vi "Decode FST200 Direction Response.vi"(10 "Direction Modbus Response":string) -> (1 "Frame Valid?":bool, 2 "Wind Direction (deg)":dbl)   [LabVIEW 2026]
panel:
  out "Direction Code Valid?":bool
  out "CRC Valid?":bool
  out "Received CRC":u16
  out "Basic Frame Valid??":bool
  out "Raw Direction Code":u16
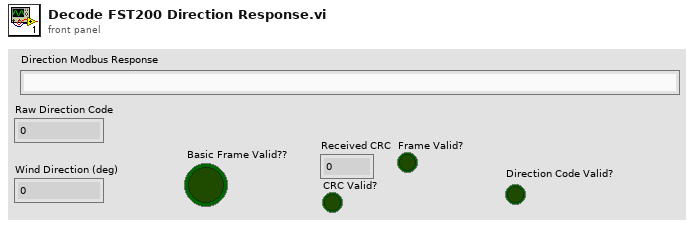
[diagram p1: front panel]
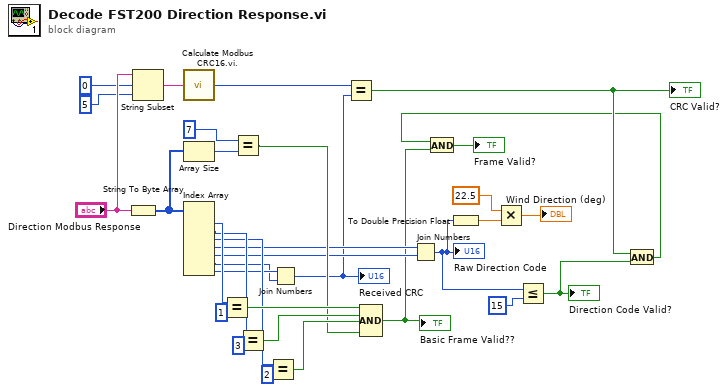
[diagram p0: block diagram]
diagram:
  n1 = String To Byte Array(string="Direction Modbus Response") -> (unsigned byte array=w33:u8[])
  n2 = String Subset(string="Direction Modbus Response", offset (0)=0, length (rest)=5 ("length (rest)")) -> (substring=w15:string)
  n3 = call "Calculate Modbus CRC16.vi..vi"("Data Bytes"=w15) -> ("Calculated CRC"=w11:u16)
  n4 = Array Size(array=w33) -> (size(s)=w32:i32)
  n5 = Index Array(array=w33) -> (element #1=w30:u8, element #2=w28:u8, element #3=w21:u8, element #4=w20:u8, element #5=w19:u8, element #6=w13:u8, element #7=w14:u8)  [unwired: 7 in]
  n6 = Equal?(x=w30, y=u8 1) -> (x = y?=w25:bool)
  n7 = Equal?(x=7, y=w32) -> (x = y?=w22:bool)
  n8 = Equal?(x=w28, y=u8 3) -> (x = y?=w24:bool)
  n9 = Equal?(x=w21, y=u8 2) -> (x = y?=w23:bool)
  n10 = Join Numbers(hi=w14, lo=w13) -> ((hi.lo)=w12:u16)
  "Received CRC" <- w12
  n11 = Equal?(x=w11, y=w12) -> (x = y?=w2:bool)
  "CRC Valid?" <- w2
  n12 = Compound Arithmetic op=AND(w25, w24, w23, w22) -> (w10:bool)
  "Basic Frame Valid??" <- w10
  n13 = Join Numbers(hi=w20, lo=w19) -> ((hi.lo)=w5:u16)
  "Raw Direction Code" <- w5
  n14 = To Double Precision Float(number=w5) -> (double precision float=w8:dbl)
  n15 = Multiply(x=22.5, y=w8) -> (x*y=→"Wind Direction (deg)":dbl)
  n16 = Less Or Equal?(x=w5, y=u16 15) -> (x <= y?=w3:bool)
  "Direction Code Valid?" <- w3
  n17 = And(x=w2, y=w3) -> (x .and. y?=w1:bool)
  n18 = And(x=w1, y=w10) -> (x .and. y?=→"Frame Valid?":bool)
